vi "loopRead.vi"() -> ()   [LabVIEW 2018]
uses:
  <vilib>/Instr/_visa.llb/VISA Configure Serial Port (Instr).vi
  <vilib>/regexp/Match Regular Expression.xnode
panel:
  out "return count 3":u32
  in  "stop":bool
  out "ID":string
  in  "Command":string="lsrs?\n"
  out "Secondary":dbl format="%^#_6e"
  out "Primary":dbl format="%^#_6e"
  out "return count 2":u32
  out "error out":errorcluster
  in  "VISA resource name":refnum<visa-resource-name>
  out "read buffer":string
  out "return count":u32
  # "Debug indicators"
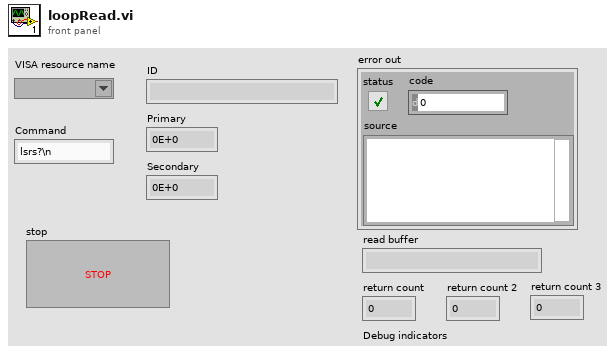
[diagram p1: front panel]
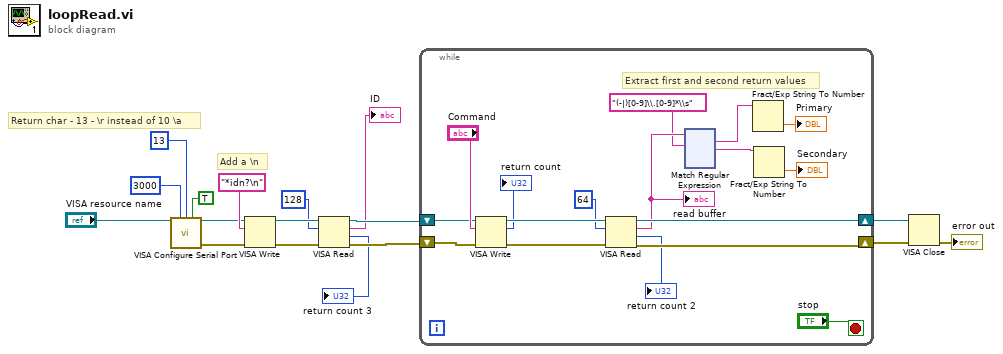
[diagram p0: block diagram]
diagram:
  # "Add a \\n"
  # "Return char - 13 - \\r instead of 10 \\a"
  n1 = call-poly "VISA Configure Serial Port"("VISA resource name"="VISA resource name", "timeout (10sec)"=u32 3000, "termination char\n(0xA = '\\n' = LF)"=u8 13 ("termination char\n(0xA = '\\n' = LF)"), "Enable Termination\nChar (T)"=TRUE ("Enable Termination\nChar (T)")) -> ("VISA resource name out"=w6:refnum<visa-resource-name>, "error out"=w5:errorcluster)  [unwired: 10 in]
  n2 = VISA Write(VISA resource name=w6, write buffer="*idn?\n" ("Command 2"), error in (no error)=w5) -> (VISA resource name out=w10:refnum<visa-resource-name>, error out=w9:errorcluster)  [unwired: 1 out]
  n3 = VISA Read(VISA resource name=w10, byte count=u32 128, error in (no error)=w9) -> (VISA resource name out=w4:refnum<visa-resource-name>, read buffer=→"ID":string, return count=→"return count 3":u32, error out=w3:errorcluster)
  n4 = while {
    shift-right: [w34] -> w14
    shift-left: w4 -> [w20]
    shift-right: [w33] -> w13
    shift-left: w3 -> [w19]
    stop <- "stop" stop-if-true
    # "Extract first and second return values"
    n5 = VISA Write(VISA resource name=w20, write buffer="Command", error in (no error)=w19) -> (VISA resource name out=w32:refnum<visa-resource-name>, return count=→"return count":u32, error out=w31:errorcluster)
    n6 = VISA Read(VISA resource name=w32, byte count=u32 64, error in (no error)=w31) -> (VISA resource name out=w34:refnum<visa-resource-name>, read buffer=w26:string, return count=→"return count 2":u32, error out=w33:errorcluster)
    "read buffer" <- w26
    n7 = xnode "Match Regular Expression"("input string"=w26, "regular expression"="(-|)[0-9]\\.[0-9]*\\s") -> ("whole match"=w24:string, "after match"=w21:string)  [unwired: 4 in, 3 out]
    n8 = Fract/Exp String To Number(string=w24) -> (number=→"Primary":dbl)  [unwired: 3 in, 1 out]
    n9 = Fract/Exp String To Number(string=w21) -> (number=→"Secondary":dbl)  [unwired: 3 in, 1 out]
  }
  n10 = VISA Close(VISA resource name=w14, error in (no error)=w13) -> (error out=→"error out":errorcluster)
